vi "Setup.vi"(8 "error in (no error)":errorcluster, 11 "TCS3472 in":refnum<class "TCS3472.lvclass">) -> (0 "error out":errorcluster, 3 "TCS3472 out":refnum<class "TCS3472.lvclass">)   [LabVIEW 2020, in "TCS3472.lvclass"]
uses:
  TCS3472.lvclass
  TCS3472.lvclass/TCS3472.ctl
  Properties/Read LINX I2C.vi
  Properties/Write LINX I2C.vi
  LINX I2C/LINX I2C.lvclass
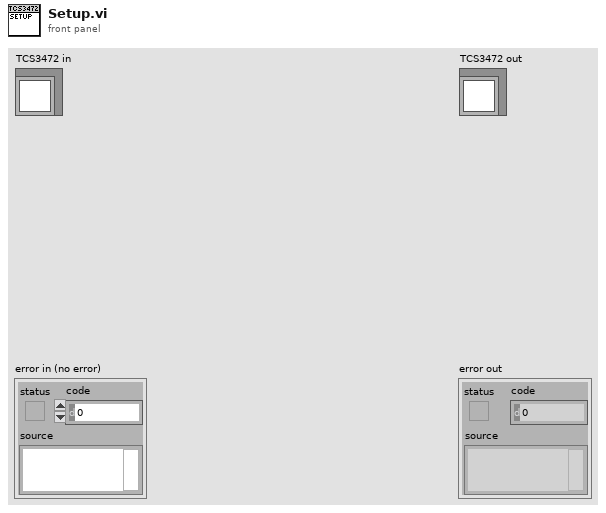
[diagram p1: front panel]
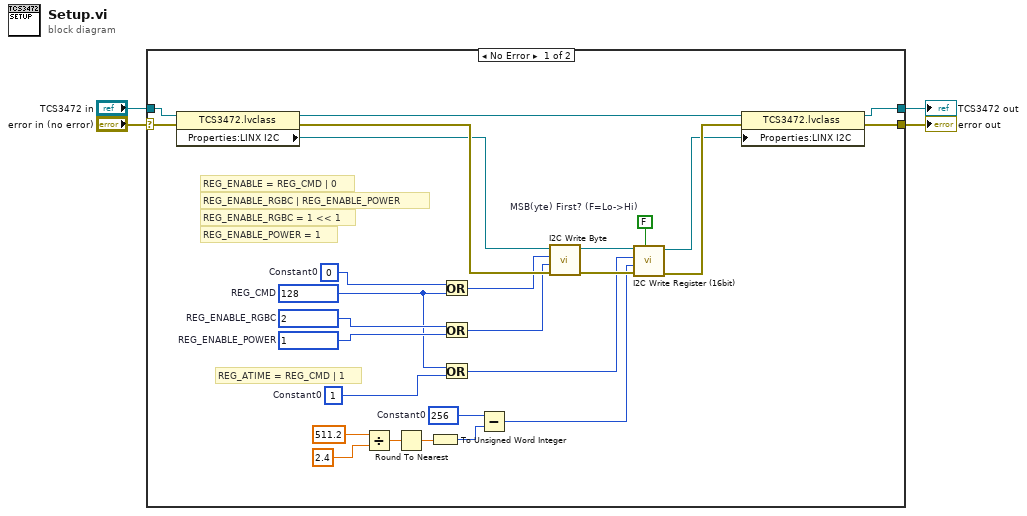
[diagram p0: block diagram]
diagram:
  n1 = case shown="No Error" "error in (no error)" {
    selector: "error in (no error)" -> [w31 w33]
    tunnel: [w28 w33] -> w3
    tunnel: [w26 w32] -> w1
    tunnel: "TCS3472 in" -> [w29 w32]
    frame No Error {
      w5 = FALSE  # MSB(yte) First? (F=Lo->Hi)
      w16 = u16 256  # Constant0
      w18 = u8 1  # Constant0
      w20 = u8 1  # REG_ENABLE_POWER
      w21 = u8 2  # REG_ENABLE_RGBC
      w23 = u8 0  # Constant0
      w17 = u8 128  # REG_CMD
      # "REG_ATIME = REG_CMD | 1"
      # "REG_ENABLE_POWER = 1"
      # "REG_ENABLE_RGBC = 1 << 1"
      # "REG_ENABLE_RGBC | REG_ENABLE_POWER"
      # "REG_ENABLE = REG_CMD | 0"
      n2 = property class="TCS3472.lvclass"(reference=w29, error in=w31) -> (reference out=w27:refnum<class "TCS3472.lvclass">, error out=w30:errorcluster, "Properties:LINX I2C"=w24:refnum<class "LINX I2C.lvclass">)
      n3 = Divide(x=511.2, y=2.4) -> (x/y=w13:dbl)
      n4 = Round To Nearest(number=w13) -> (nearest integer value=w12:dbl)
      n5 = To Unsigned Word Integer(number=w12) -> (unsigned 16bit integer=w11:u16)
      n6 = Or(x=w23, y=w17) -> (x .or. y?=w22:u8)
      n7 = Or(x=w21, y=w20) -> (x .or. y?=w19:u8)
      n8 = Or(x=w17, y=w18) -> (x .or. y?=w7:u8)
      n9 = Subtract(x=w16, y=w11) -> (x-y=w6:u16)
      n10 = call "I2C Write Byte.vi"("error in (no error)"=w30, "Value"=w19, "Register Address"=w22, "LINX I2C in"=w24) -> ("error out"=w25:errorcluster, "LINX I2C out"=w9:refnum<class "LINX I2C.lvclass">)  [unwired: 6 in]
      n11 = call "I2C Write Register (16bit).vi"("MSB(yte) First? (F=Lo->Hi)"=w5, "error in (no error)"=w25, "Value"=w6, "Register Address"=w7, "LINX I2C in"=w9) -> ("error out"=w10:errorcluster, "LINX I2C out"=w8:refnum<class "LINX I2C.lvclass">)  [unwired: 5 in]
      n12 = property class="TCS3472.lvclass"(reference=w27, error in=w10, "Properties:LINX I2C"=w8) -> (reference out=w26:refnum<class "TCS3472.lvclass">, error out=w28:errorcluster)
    }
    frame Error {
    }
  }
  "error out" <- w3
  "TCS3472 out" <- w1
